vi "Error Manager (Main).vi"(8 "Error In":errorcluster, 11 "Settings Filepath":path) -> (0 "Error Out":errorcluster)   [LabVIEW 2016, in "Error Manager.lvlib"]
doc: "This is the main VI of the Error Manager module.\n\nThe Error Manager is a stand-alone, asynchronous LabVIEW module that can help log LabVIEW errors to file, display error details to the user, and display the chronological or inverse-chronological list of errors that occurred since the module started. The module is framework-agnostic, reusable from project to project, and can keep working even when being \"spammed\" with many instances of the same error (spam protection functionality). Using the Error Manager in a new application helps ensure out-of-the-box robust and reliable error handling.\n\nCopyright (c) 2023, Robusto Systems Ltd (UK)"
uses:
  Error Manager.lvlib
  <vilib>/Utility/error.llb/DialogType.ctl
  Private VIs/Read-Unread Status (enum).ctl
  Private VIs/Reported Error (cluster).ctl
  Multi-Column Listbox/MCL.lvclass
  Error Log/Error Log.lvclass
  Display Order Combo Box/Display Order Combo Box.lvclass
  Queues/MHL Queue/MHL Queue.lvclass
  Queues/MHL Queue/Command (enum).ctl
  Private VIs/Error in current one-second interval (cluster).ctl
  Queues/Log To File Loop Queue/Log To File Loop Queue.lvclass
  Queues/Log To File Loop Queue/Command (enum).ctl
  Error Log/Error Type (enum).ctl
  Error Log/Error to be logged (cluster).ctl
  Queues/New Error Window Loop Queue/Error Window Loop Queue.lvclass
  Queues/New Error Window Loop Queue/Command (enum).ctl
  Error Display Window/Error Display Window.lvclass
  Error Display Window/Error Details (cluster).ctl
  Private VIs/GUI Object References (cluster).ctl
  Mark Selected Errors As Read Button/Mark Selected Errors As Read Button.lvclass
  Mark All Errors As Read Button/Mark All Errors As Read Button.lvclass
  Settings/Settings.lvclass
  Public API VIs/Show Error Window Instruction (enum).ctl
panel:
  out "Module Init Timestamp":timestamp
  out "Read Settings Error":errorcluster
  out "Are All Errors Read?":bool
  out "MCL NewVal":i32[](array[numeric])
  in  "Mark All Errors As Read":bool
  in  "Mark Selected Errors As Read":bool
  out "Metronome Loop iteration":i32
  out "\"New Error Window\" Loop iteration":i32
  out "\"Log to File\" Loop iteration":i32
  out "\"Handle Error\" Error":errorcluster
  in  "Sizing Tool":bool
  in  "Display Order ComboBox":string(combo) caption="Display Order"
  out "Close Module Error":errorcluster
  in  "Open Error Logs Folder":bool
  in  "Open Error Log in Notepad":bool
  out "Error Log Filepath":string
  out "Full Error Message":string caption="Error Message Of Selected Error"
  in  "MCL":i32[](listbox) caption="Errors"
  out "Close Module?":bool
  out "EHL iteration":i32
  out "MHL iteration":i32
  out "Initialisation Error":errorcluster
  # "Error Manager\nThis is the main VI of the Error Manager module."
  # "The region below is invisible to the user. For developer use only."
  # "Input\nInputs to the VI"
  # "Development\ncontrols/indicators useful for development and testing, but which are not outputs of the VI"
  # "Output\nOutputs of the VI"
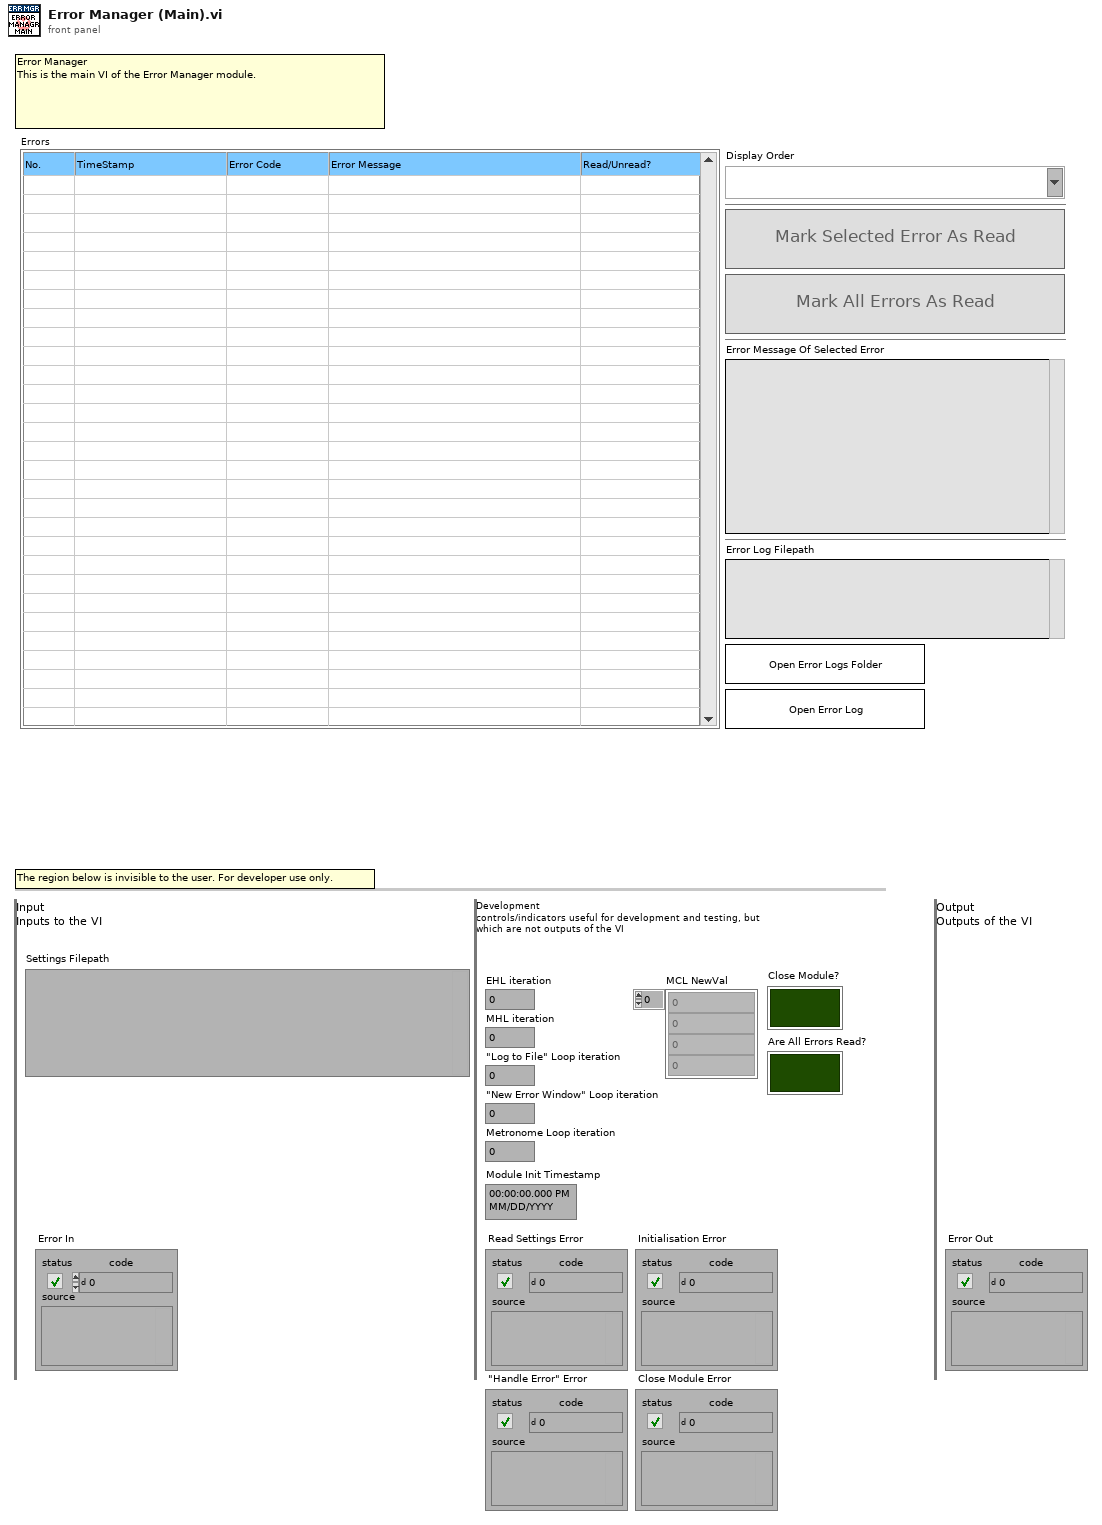
[diagram p1: front panel]
types:
  T1 = typedef "Error Manager.lvlib/MHL Queue.lvclass/Command (enum).ctl" = enum16{"Init Module", "Close Module", "Internal Error", "Create Error Log File", "Show Front Panel", "Handle Error", "Refresh MCL", "MCL Value Change", "Change Display Order", "One-Second Interval Expired", "Mark Selected Errors As Read", "Mark All Errors As Read", "Refresh Button State - MSEAR", "Refresh Button State - MAEAR"}
  T2 = typedef "Error Manager.lvlib/Error Window Loop Queue.lvclass/Command (enum).ctl" = enum16{"Init Loop", "Close Loop", "Show Error Window"}
  T3 = typedef "Error Manager.lvlib/Log To File Loop Queue.lvclass/Command (enum).ctl" = enum16{"Init Loop", "Close Loop", "Log Error"}
  T4 = typedef "Error Manager.lvlib/Read-Unread Status (enum).ctl" = enum16{"Unread", "Read"}
  T5 = typedef "Error Manager.lvlib/GUI Object References (cluster).ctl" = cluster{"MCL":refnum<vi>, "Display Order ComboBox":refnum<vi>, "Mark Selected Errors As Read":refnum<vi>, "Mark All Errors As Read":refnum<vi>, "Full Error Message":refnum<vi>, "Error Log Filepath":refnum<vi>, "Open Error Logs Folder":refnum<vi>, "Open Error Log in Notepad":refnum<vi>}
  T6 = typedef "Error Manager.lvlib/Module Data (cluster).ctl" = cluster{"GUI Object References":T5, "Total no. of errors reported":i32, "Total no. of errors handled":i32, "Handled Errors (chronological order)":T7[], "Display Order":T8, "Errors in current one-second interval":T9[], "Module Init Timestamp":timestamp, "Module Close Timestamp":timestamp}
  T7 = typedef "Error Manager.lvlib/Handled Error (cluster).ctl" = cluster{"Error Number":i32, "Timestamp":timestamp, "Error code":i32, "Error message":string, "Read-Unread Status":T4}
  T8 = typedef "Error Manager.lvlib/Display Order (enum).ctl" = enum16{"Most Recent First (inverse-chronological)", "Oldest First (chronological)"}
  T9 = typedef "Error Manager.lvlib/Error in current one-second interval (cluster).ctl" = cluster{"Error code":i32, "No. of times error reported":u32, "No. of times error handled":u32}
  T10 = typedef "Error Manager.lvlib/Settings.lvclass/Error_Log_Setting (enum).ctl" = enum16{"Log Full Error Details", "Log Error Codes Only", "Do Not Log"}
  T11 = typedef "Error Manager.lvlib/Settings.lvclass/Window_Behaviour (enum).ctl" = enum16{"Default", "Floating", "Modal"}
  T12 = typedef "Error Manager.lvlib/Reported Error (cluster).ctl" = cluster{"Error Timestamp":timestamp, "Error Code":i32, "Error message":string, "Show Error Window?":T13}
  T13 = typedef "Error Manager.lvlib/Show Error Window Instruction (enum).ctl" = enum16{"Use Default Setting", "Show", "Do Not Show"}
  T14 = typedef "Error Manager.lvlib/Error Log.lvclass/Error to be logged (cluster).ctl" = cluster{"Error Type":T15, "Error Number":i32, "Error Timestamp":timestamp, "Error code":i32, "Error message":string}
  T15 = typedef "Error Manager.lvlib/Error Log.lvclass/Error Type (enum).ctl" = enum16{"New", "Identical to last logged error"}
  T16 = typedef "Error Manager.lvlib/Settings.lvclass/Show_Error_Window_Default (enum).ctl" = enum16{"Show For All Errors", "Show For New Errors", "Show For New Error Codes", "Do Not Show"}
  T17 = typedef "Error Manager.lvlib/Error Display Window.lvclass/Error Details (cluster).ctl" = cluster{"Error Code":i32, "Error Message":string, "Error Timestamp":timestamp}
  T18 = typedef "DialogType.ctl" = u16
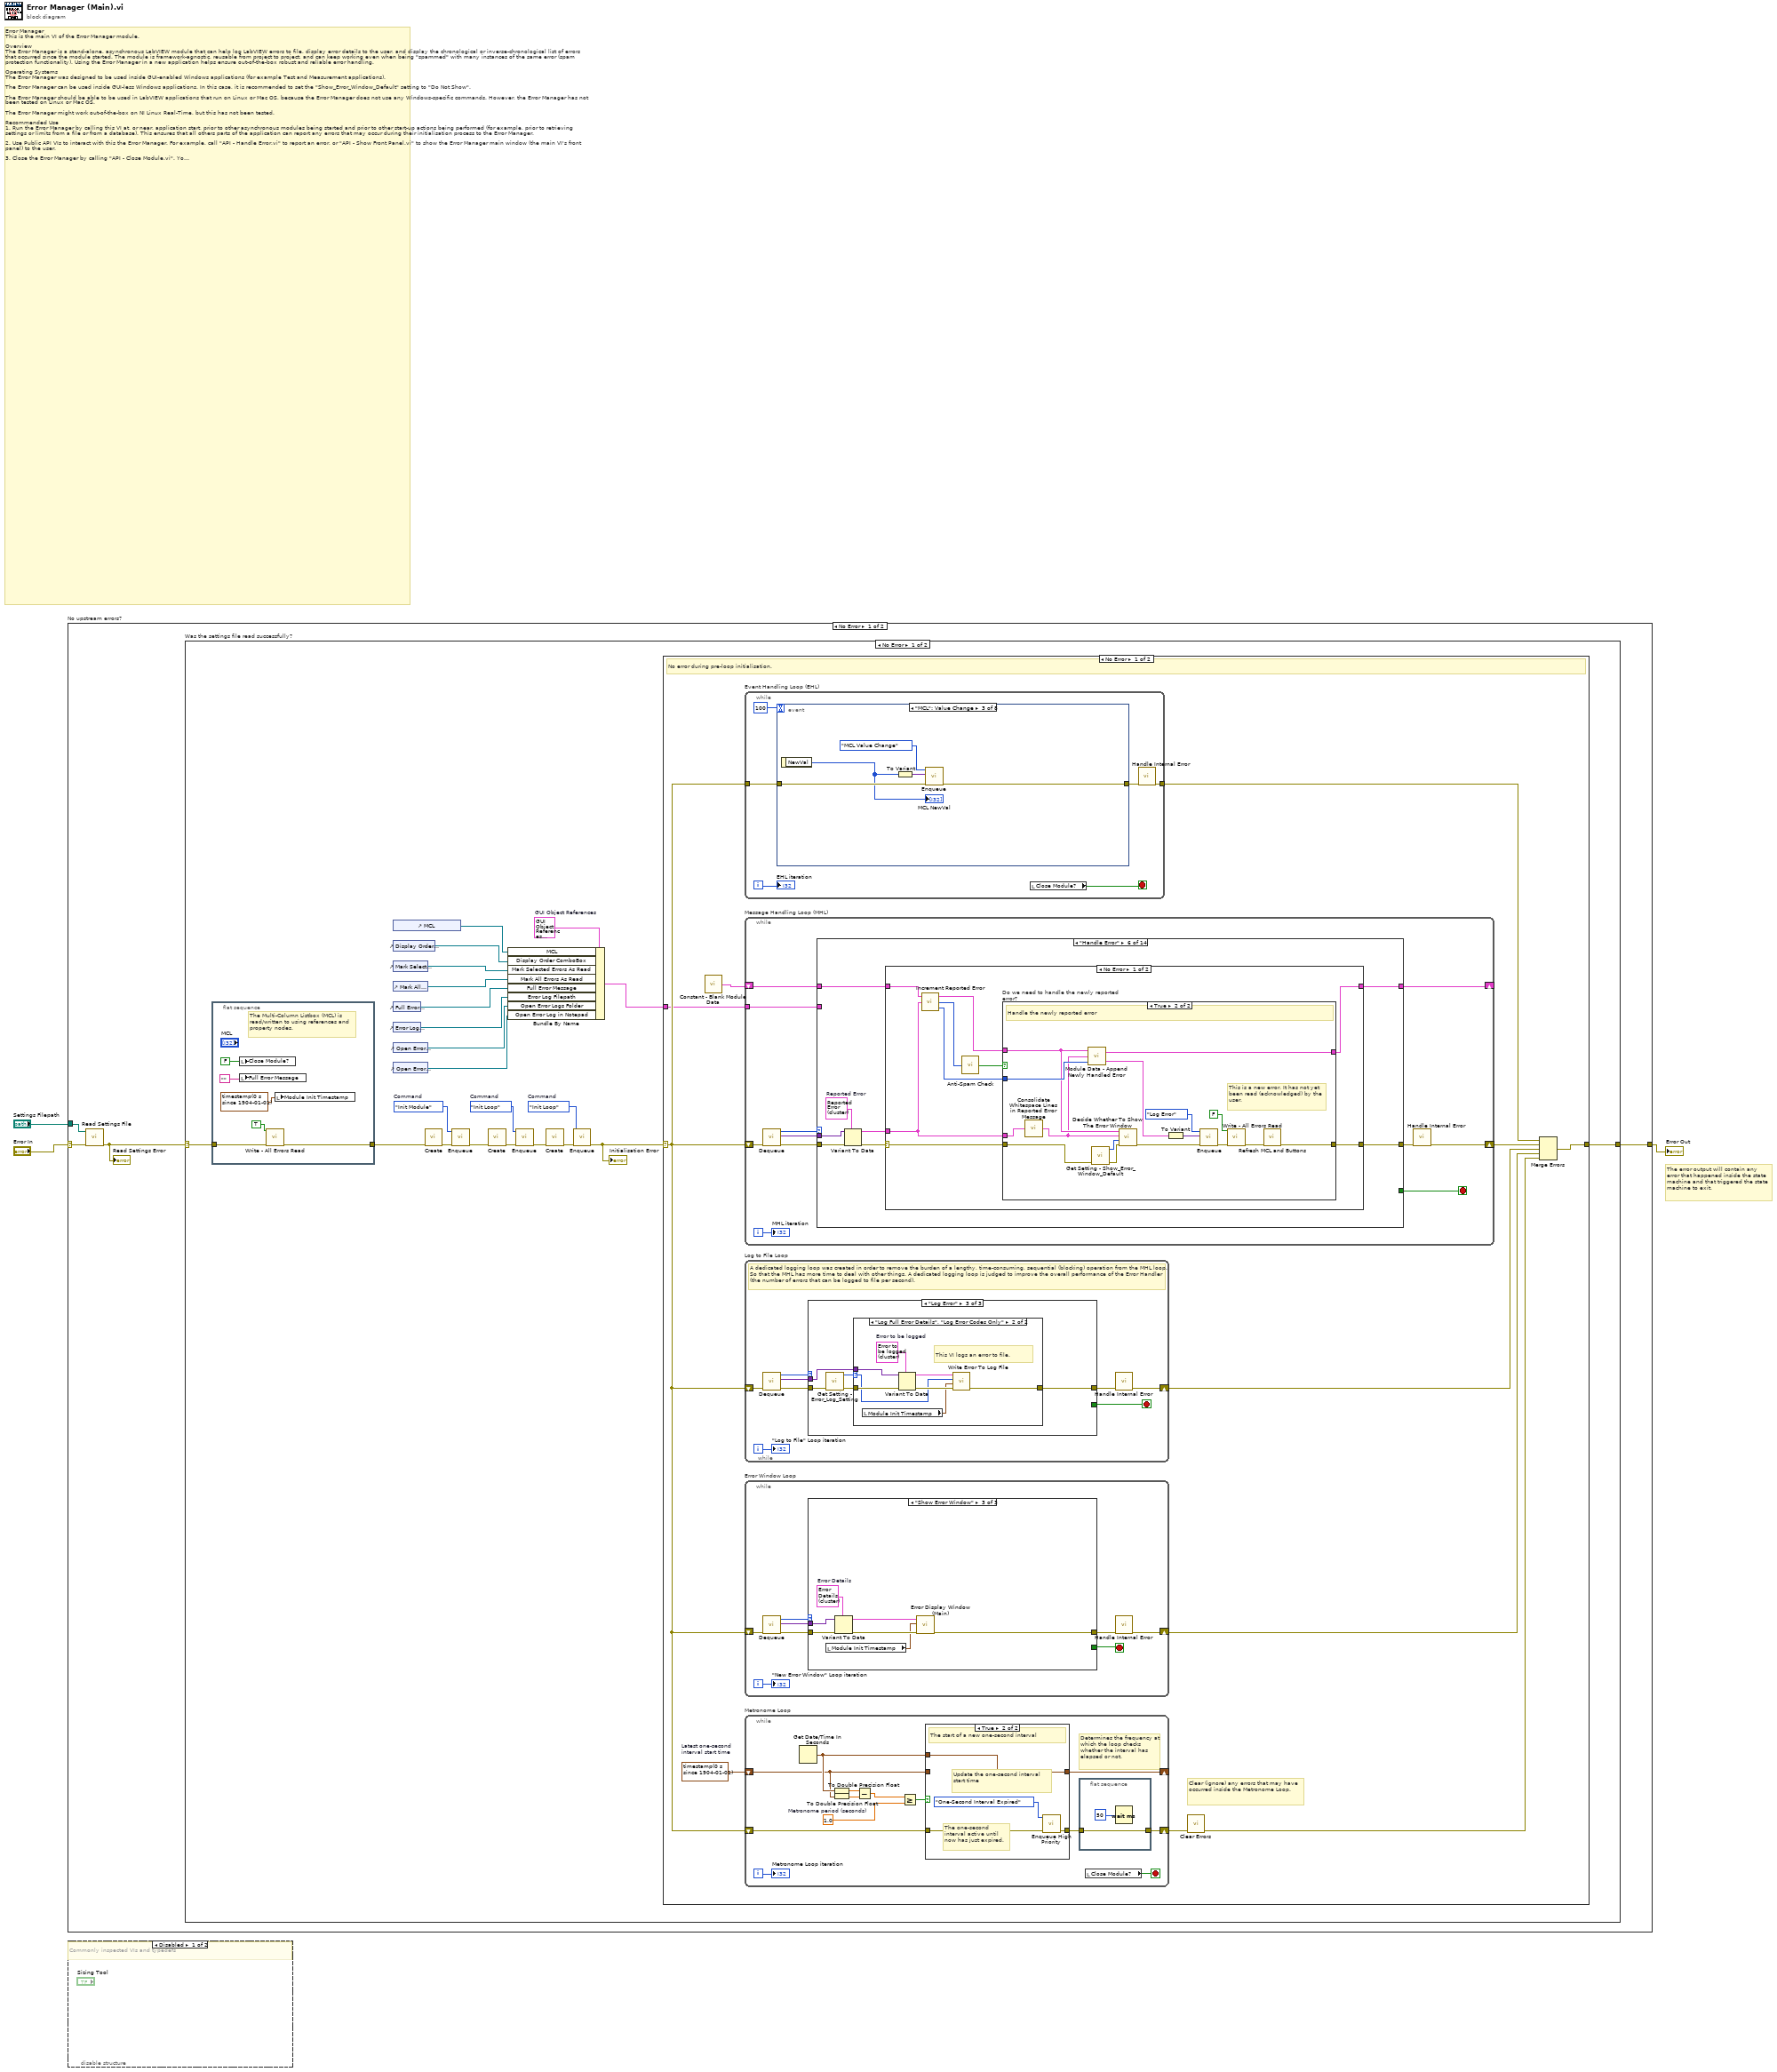
[diagram p0: block diagram]
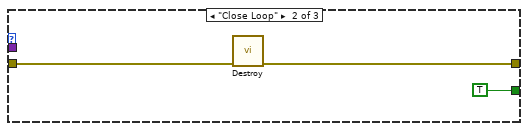
[diagram p3: hidden frame]
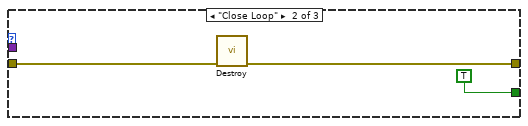
[diagram p5: hidden frame]
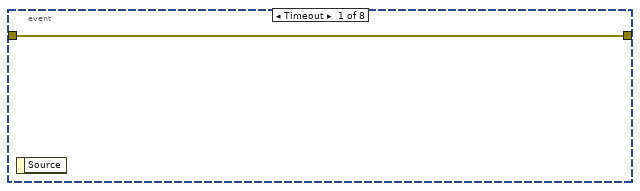
[diagram p7: hidden frame]
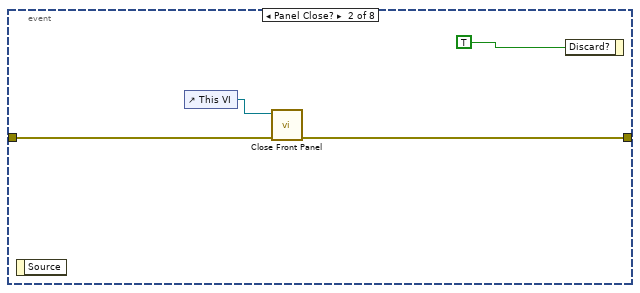
[diagram p8: hidden frame]
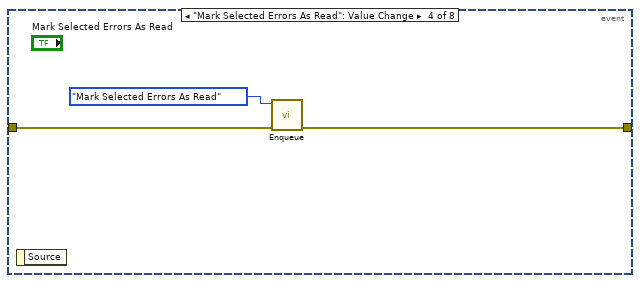
[diagram p9: hidden frame]
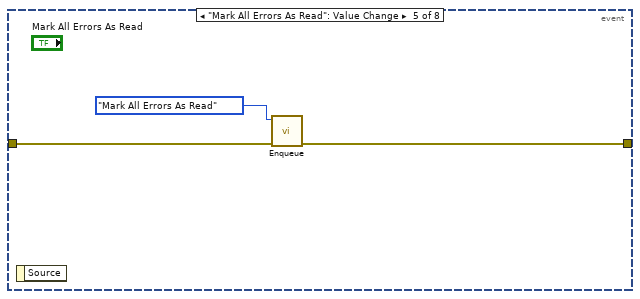
[diagram p10: hidden frame]
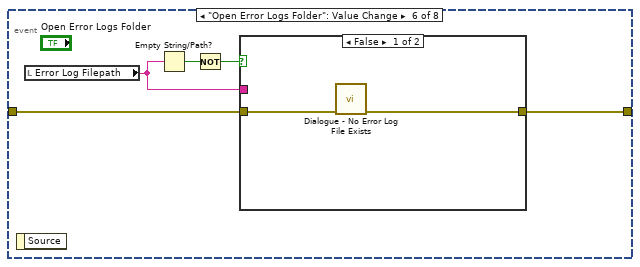
[diagram p11: hidden frame]
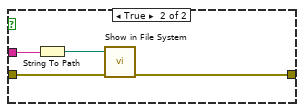
[diagram p12: hidden frame]
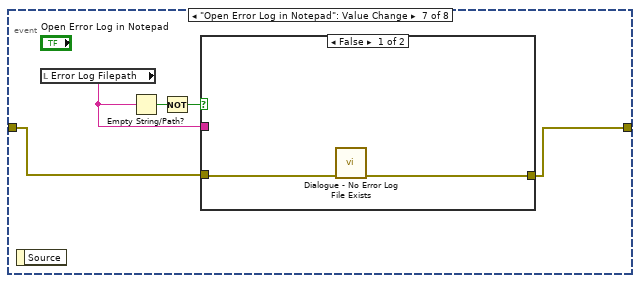
[diagram p13: hidden frame]
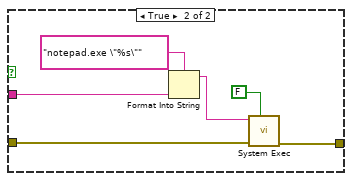
[diagram p14: hidden frame]
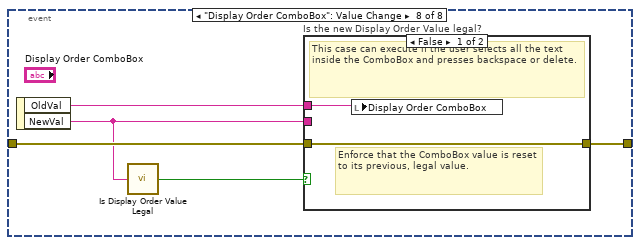
[diagram p15: hidden frame]
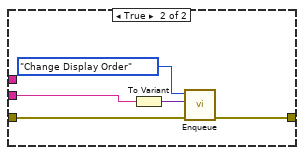
[diagram p16: hidden frame]
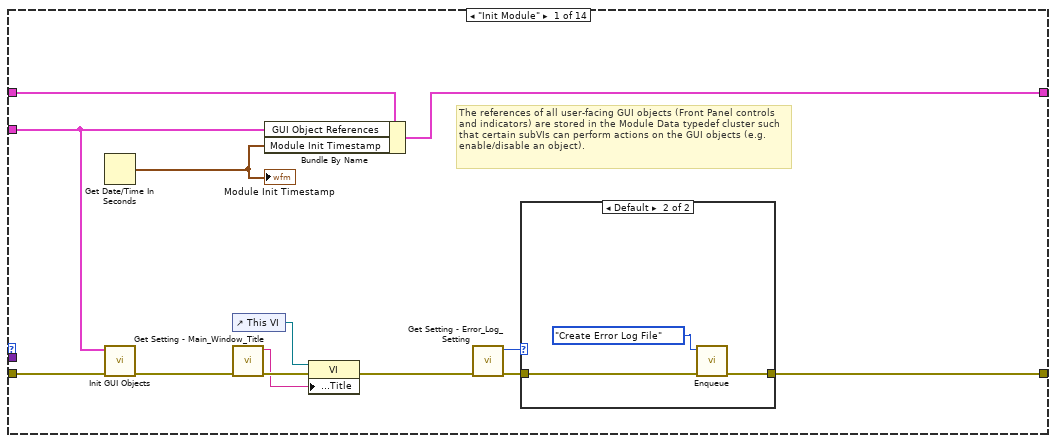
[diagram p17: hidden frame]
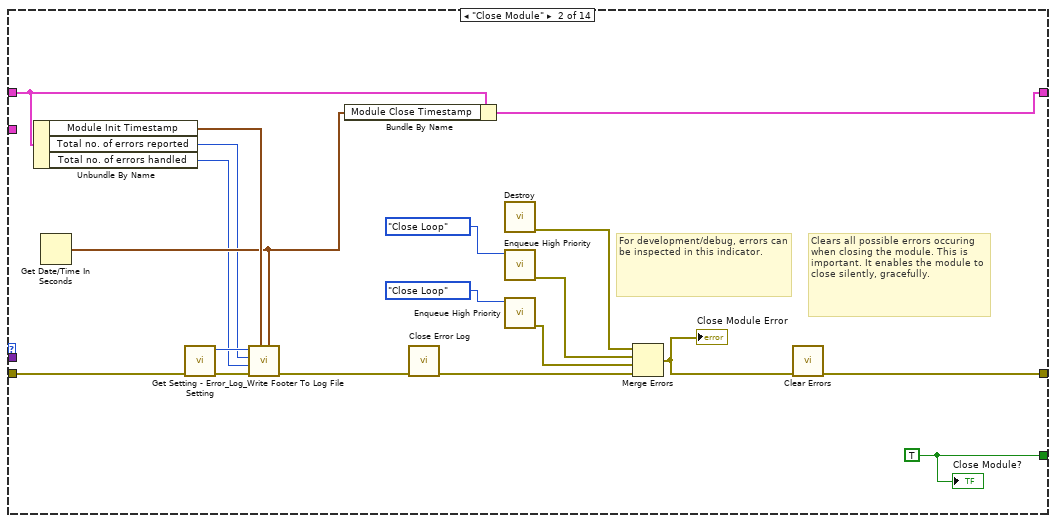
[diagram p19: hidden frame]
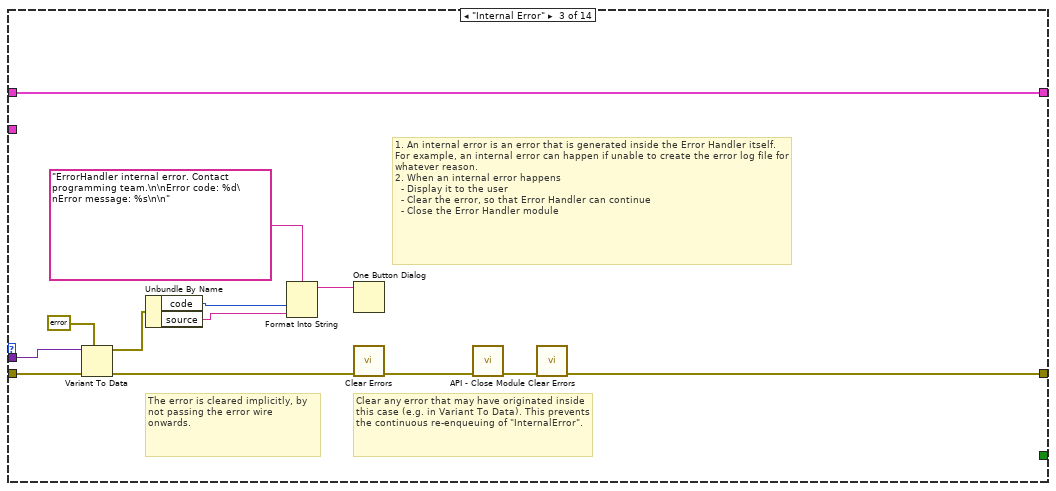
[diagram p20: hidden frame]
diagram:
  # "Error Manager\nThis is the main VI of the Error Manager module.\n\nOverview\nThe Error Manager is a stand-alone, asynchronous LabVIEW module that can help log LabVIEW errors to file, display error details to the user, and display the chronological or inverse-chronological list of errors that occurred since the module started. The module is framework-agnostic, reusable from project to project, and can keep working even when being \"spammed\" with many instances of the same error (spam protection functionality). Using the Error Manager in a new application helps ensure out-of-the-box robust and reliable error handling.\n\nOperating Systems\nThe Error Manager was designed to be used inside GUI-enabled Windows applications (for example Test and Measurement applications).\n\nThe Error Manager can be used inside GUI-less Windows applications. In this case, it is recommended to set the \"Show_Error_Window_Default\" setting to \"Do Not Show\".\n\nThe Error Manager should be able to be used in LabVIEW applications that run on Linux or Mac OS, because the Error Manager does not use any Windows-specific commands. However, the Error Manager has not been tested on Linux or Mac OS.\n\nThe Error Manager might work out-of-the-box on NI Linux Real-Time, but this has not been tested.\n\nRecommended Use\n1. Run the Error Manager by calling this VI at, or near, application start, prior to other asynchronous modules being started and prior to other start-up actions being performed (for example, prior to retrieving settings or limits from a file or from a database). This ensures that all others parts of the application can report any errors that may occur during their initialisation process to the Error Manager.\n\n2. Use Public API VIs to interact with this the Error Manager. For example, call \"API - Handle Error.vi\" to report an error, or \"API - Show Front Panel.vi\" to show the Error Manager main window (the main VI's front panel) to the user.\n\n3. Close the Error Manager by calling \"API - Close Module.vi\". You can close the Error Manager module at any time you like, but it is recommended to close Error Manager during app shutdown, after all other shutdown operations have been completed (for example, after all other asynchronous modules have been stopped). This enables the Error Manager to log any errors that may occur during app shutdown.\n\nPublic GitHub Repository: https://github.com/RobustoSystems/ErrorManager \n\nSuggestions\nPlease email us at engineering@robustosystems.com with any bug reports or suggestions. Alternatively, feel free to create a new issue in the public GitHub repository.\n\nEULA\nThe Error Manager is free and open-source, and is published under the MIT license, which is one of the most permissive types of licenses. You can use the Error Manager inside commercial, closed-source applications.\n\nMIT License\n\nCopyright (c) 2023, Robusto Systems Ltd (UK)\n\nPermission is hereby granted, free of charge, to any person obtaining a copy\nof this software and associated documentation files (the \"Software\"), to deal\nin the Software without restriction, including without limitation the rights\nto use, copy, modify, merge, publish, distribute, sublicense, and/or sell\ncopies of the Software, and to permit persons to whom the Software is\nfurnished to do so, subject to the following conditions:\n\nThe above copyright notice and this permission notice shall be included in all\ncopies or substantial portions of the Software.\n\nTHE SOFTWARE IS PROVIDED \"AS IS\", WITHOUT WARRANTY OF ANY KIND, EXPRESS OR\nIMPLIED, INCLUDING BUT NOT LIMITED TO THE WARRANTIES OF MERCHANTABILITY,\nFITNESS FOR A PARTICULAR PURPOSE AND NONINFRINGEMENT. IN NO EVENT SHALL THE\nAUTHORS OR COPYRIGHT HOLDERS BE LIABLE FOR ANY CLAIM, DAMAGES OR OTHER\nLIABILITY, WHETHER IN AN ACTION OF CONTRACT, TORT OR OTHERWISE, ARISING FROM,\nOUT OF OR IN CONNECTION WITH THE SOFTWARE OR THE USE OR OTHER DEALINGS IN THE\nSOFTWARE."
  # "The error output will contain any error that happened inside the state machine and that triggered the state machine to exit."
  n1 = case "No upstream errors?" shown="No Error" "Error In" {
    selector: "Error In" -> [w6 w419]
    tunnel: [w7 w419] -> w3
    tunnel: "Settings Filepath" -> [w5 _]
    frame No Error {
      n2 = call "Read Settings File.vi"("error in (no error)"=w6, "Settings Filepath"=w5) -> ("error out"=w4:errorcluster)  [unwired: 9 in]
      "Read Settings Error" <- w4
      n3 = case "Was the settings file read successfully?" shown="No Error" w4 {
        selector: w4 -> [w8 w417]
        tunnel: [w29 w416] -> w7
        frame No Error {
          w18 = T5 {"MCL"=refnum, "Display Order ComboBox"=refnum, "Mark Selected Errors As Read"=refnum, "Mark All Errors As Read"=refnum, "Full Error Message"=refnum, "Error Log Filepath"=refnum, "Open Error Logs Folder"=refnum, "Open Error Log in Notepad"=refnum}  # GUI Object References
          w20 = Command_(enum)."Init Loop"  # Command
          w23 = Command_(enum)."Init Loop"  # Command
          w26 = Command_(enum)."Init Module"  # Command
          n4 = flat-sequence {
            tunnel: [w34] -> w19
            tunnel: w8 -> [w33]
            frame #0 {
              # "The Multi-Column Listbox (MCL) is read/written to using references and property nodes."
              n5 = local write "Close Module?"(FALSE ("Close module?")) -> ()
              n6 = local write "Full Error Message"("") -> ()
              n7 = call "Write - All Errors Read.vi"("error in (no error)"=w33, "All Errors Read?"=TRUE) -> ("error out"=w34:errorcluster)  [unwired: 9 in]
              n8 = local write "Module Init Timestamp"(timestamp(0 s since 1904-01-01) ("Module Init Timestamp")) -> ()
            }
          }
          n9 = control-ref of="MCL"() -> (w17:refnum<vi>)
          n10 = control-ref of="Display Order ComboBox"() -> (w16:refnum<vi>)
          n11 = control-ref of="Mark Selected Errors As Read"() -> (w15:refnum<vi>)
          n12 = control-ref of="Mark All Errors As Read"() -> (w14:refnum<vi>)
          n13 = control-ref of="Full Error Message"() -> (w13:refnum<vi>)
          n14 = control-ref of="Error Log Filepath"() -> (w12:refnum<vi>)
          n15 = control-ref of="Open Error Logs Folder"() -> (w11:refnum<vi>)
          n16 = control-ref of="Open Error Log in Notepad"() -> (w10:refnum<vi>)
          n17 = call "Create.vi"("error in (no error)"=w19) -> ("error out"=w28:errorcluster)  [unwired: 10 in]
          n18 = call "Enqueue.vi"("error in (no error)"=w28, "Command"=w26) -> ("error out"=w27:errorcluster)  [unwired: 9 in]
          n19 = call "Create.vi"("error in (no error)"=w27) -> ("error out"=w25:errorcluster)  [unwired: 10 in]
          n20 = Bundle By Name(cluster=w18, "MCL"=w17, "Display Order ComboBox"=w16, "Mark Selected Errors As Read"=w15, "Mark All Errors As Read"=w14, "Full Error Message"=w13, "Error Log Filepath"=w12, "Open Error Logs Folder"=w11, "Open Error Log in Notepad"=w10) -> (w9:T5)
          n21 = call "Enqueue.vi"("error in (no error)"=w25, "Command"=w23) -> ("error out"=w24:errorcluster)  [unwired: 9 in]
          n22 = call "Create.vi"("error in (no error)"=w24) -> ("error out"=w22:errorcluster)  [unwired: 10 in]
          n23 = call "Enqueue.vi"("error in (no error)"=w22, "Command"=w20) -> ("error out"=w21:errorcluster)  [unwired: 9 in]
          "Initialisation Error" <- w21
          n24 = case shown="No Error" w21 {
            selector: w21 -> [w39 w415]
            tunnel: [w45 w414] -> w29
            tunnel: w9 -> [w36 _]
            frame No Error {
              w43 = timestamp(0 s since 1904-01-01)  # Latest one-second interval start time
              # "Clear (ignore) any errors that may have occurred inside the Metronome Loop."
              # "No error during pre-loop initialisation."
              n25 = call "Constant - Blank Module Data.vi"() -> ("Blank Module Data"=w41:T6)
              n26 = while "Event Handling Loop (EHL)" {
                tunnel: w39 -> [w94]
                tunnel: [w92] -> w44
                i -> [w97]
                stop <- w95 stop-if-true
                n27 = event shown="[2] \"MCL\": Value Change" {
                  selector: _ -> [_ _ _ _ _ _ _ _]
                  dyn-events: _ -> [_ _ _ _ _ _ _ _]
                  timeout: 100 -> [_ _ _ _ _ _ _ _]
                  tunnel: w94 -> [w98 w100 w107 w110 w113 w115 w126 w142]
                  tunnel: [w98 w99 w106 w109 w112 w114 w125 w141] -> w93
                  event Timeout {
                    n28 = event-data() -> ()  [unwired: 1 in, 1 out]
                  }
                  event Panel Close? {
                    n29 = event-data() -> ()  [unwired: 1 in, 1 out]
                    n30 = control-ref of="This VI"() -> (w101:refnum<vi>)
                    n31 = call "Close Front Panel.vi"("Error In"=w100, "VI Reference"=w101) -> ("Error Out"=w99:errorcluster)  [unwired: 9 in]
                    n32 = event-data("Discard?"=TRUE) -> ()  [unwired: 1 in, 1 out]
                  }
                  event "MCL": Value Change {
                    n33 = event-data() -> ("NewVal"=w104:i32[])  [unwired: 1 in]
                    "MCL NewVal" <- w104
                    n34 = To Variant(anything=w104) -> (Variant=w103:variant)
                    n35 = call "Enqueue.vi"("error in (no error)"=w107, "Data"=w103, "Command"=Command_(enum)."MCL Value Change") -> ("error out"=w106:errorcluster)  [unwired: 8 in]
                  }
                  event "Mark Selected Errors As Read": Value Change {
                    n36 = event-data() -> ()  [unwired: 1 in, 1 out]
                    n37 = call "Enqueue.vi"("error in (no error)"=w110, "Command"=Command_(enum)."Mark Selected Errors As Read") -> ("error out"=w109:errorcluster)  [unwired: 9 in]
                  }
                  event "Mark All Errors As Read": Value Change {
                    n38 = event-data() -> ()  [unwired: 1 in, 1 out]
                    n39 = call "Enqueue.vi"("error in (no error)"=w113, "Command"=Command_(enum)."Mark All Errors As Read") -> ("error out"=w112:errorcluster)  [unwired: 9 in]
                  }
                  event "Open Error Logs Folder": Value Change {
                    n40 = event-data() -> ()  [unwired: 1 in, 1 out]
                    n41 = local read "Error Log Filepath"() -> (w116:string)
                    n42 = Empty String/Path?(string/path=w116) -> (empty?=w118:bool)
                    n43 = Not(x=w118) -> (.not. x?=w117:bool)
                    n44 = case shown="False" w117 {
                      tunnel: w116 -> [_ w123]
                      tunnel: w115 -> [w119 w122]
                      tunnel: [w120 w121] -> w114
                      frame False {
                        n45 = call "Dialogue - No Error Log File Exists.vi"("error in (no error)"=w119) -> ("error out"=w120:errorcluster)  [unwired: 10 in]
                      }
                      frame True {
                        n46 = String To Path(string=w123) -> (path=w124:path)
                        n47 = call <vilib>:"Show in File System.vi"("error in (no error)"=w122, "file or directory path"=w124) -> ("error out"=w121:errorcluster)  [unwired: 9 in]
                      }
                    }
                  }
                  event "Open Error Log in Notepad": Value Change {
                    n48 = event-data() -> ()  [unwired: 1 in, 1 out]
                    n49 = local read "Error Log Filepath"() -> (w127:string)
                    n50 = Empty String/Path?(string/path=w127) -> (empty?=w128:bool)
                    n51 = Not(x=w128) -> (.not. x?=w129:bool)
                    n52 = case shown="False" w129 {
                      tunnel: w126 -> [w131 w135]
                      tunnel: [w130 w134] -> w125
                      tunnel: w127 -> [_ w133]
                      frame False {
                        n53 = call "Dialogue - No Error Log File Exists.vi"("error in (no error)"=w131) -> ("error out"=w130:errorcluster)  [unwired: 10 in]
                      }
                      frame True {
                        n54 = Format Into String(format string="notepad.exe \"%s\"", w133) -> (resulting string=w136:string)  [unwired: 2 in, 1 out]
                        n55 = call <vilib>:"System Exec.vi"("wait until completion? (T)"=FALSE, "error in (no error)"=w135, "command line"=w136) -> ("error out"=w134:errorcluster)  [unwired: 5 in, 3 out]
                      }
                    }
                  }
                  event "Display Order ComboBox": Value Change {
                    n56 = event-data() -> ("OldVal"=w138:string, "NewVal"=w140:string)  [unwired: 1 in]
                    n57 = call "Is Display Order Value Legal.vi"("New Display Order Value"=w140) -> ("Is Display Order Value Legal?"=w139:bool)
                    n58 = case "Is the new Display Order Value legal?" shown="False" w139 {
                      tunnel: w142 -> [w144 w149]
                      tunnel: [w144 w148] -> w141
                      tunnel: w140 -> [_ w145]
                      tunnel: w138 -> [w143 _]
                      frame False {
                        # "Enforce that the ComboBox value is reset to its previous, legal value."
                        # "This case can execute if the user selects all the text inside the ComboBox and presses backspace or delete."
                        n59 = local write "Display Order ComboBox"(w143) -> ()
                      }
                      frame True {
                        n60 = To Variant(anything=w145) -> (Variant=w147:variant)
                        n61 = call "Enqueue.vi"("error in (no error)"=w149, "Data"=w147, "Command"=Command_(enum)."Change Display Order") -> ("error out"=w148:errorcluster)  [unwired: 8 in]
                      }
                    }
                  }
                }
                n62 = local read "Close Module?"() -> (w95:bool)
                n63 = call "Handle Internal Error.vi"("error in (no error)"=w93) -> ("error out"=w92:errorcluster)  [unwired: 10 in]
                "EHL iteration" <- w97
              }
              n64 = while "Message Handling Loop (MHL)" {
                shift-right: [w154] -> w46
                shift-left: w39 -> [w158]
                shift-right: [w156] -> _
                shift-left: w41 -> [w151]
                tunnel: w36 -> [w150]
                i -> [w157]
                stop <- w160 stop-if-true
                n65 = call "Dequeue.vi"("error in (no error)"=w158) -> ("error out"=w159:errorcluster, "Data"=w152:variant, "Command"=w153:T1)  [unwired: 8 in]
                n66 = case shown="\"Handle Error\"" w153 {
                  tunnel: w159 -> [w169 w185 w206 w213 w229 w243 w278 w291 w310 w323 w338 w352 w381 w391]
                  tunnel: [w173 w194 w197 w215 w234 w240 w277 w284 w305 w322 w334 w342 w379 w389] -> w155
                  tunnel: [_ w195 _ _ _ _ _ _ _ _ _ _ _ _] -> w160
                  tunnel: w152 -> [_ _ w204 _ _ w241 _ w287 w301 _ _ _ _ _]
                  tunnel: w151 -> [w168 w182 w202 w211 w235 w237 w281 w290 w303 w319 w336 w349 w383 w388]
                  tunnel: [w167 w183 w202 w211 w235 w238 w281 w290 w304 w320 w335 w348 w383 w388] -> w156
                  tunnel: w150 -> [w166 _ _ _ _ _ _ _ _ _ _ _ _ _]
                  frame "Init Module" {
                    # "The references of all user-facing GUI objects (Front Panel controls and indicators) are stored in the Module Data typedef cluster such that certain subVIs can perform actions on the GUI objects (e.g. enable/disable an object)."
                    n67 = Get Date/Time In Seconds() -> (seconds since 1Jan1904=w161:timestamp)
                    "Module Init Timestamp" <- w161
                    n68 = call "Init GUI Objects.vi"("Error In"=w169, "GUI Object References"=w166) -> ("Error Out"=w170:errorcluster)  [unwired: 9 in]
                    n69 = control-ref of="This VI"() -> (w171:refnum<vi>)
                    n70 = call "Get Setting - Main_Window_Title.vi"("Error In"=w170) -> ("Error Out"=w165:errorcluster, "Main_Window_Title"=w164:string)  [unwired: 9 in]
                    n71 = Bundle By Name(cluster=w168, "GUI Object References"=w166, "Module Init Timestamp"=w161) -> (w167:T6)
                    n72 = property class="VI"(reference=w171, error in=w165, "Front Panel.Title"=w164) -> (error out=w172:errorcluster)  [unwired: 1 out]
                    n73 = call "Get Setting - Error_Log_Setting.vi"("Error In"=w172) -> ("Error Out"=w163:errorcluster, "Error_Log_Setting"=w162:T10)  [unwired: 9 in]
                    n74 = case shown="Default" w162 {
                      tunnel: [w174 w177] -> w173
                      tunnel: w163 -> [w174 w175]
                      frame "Do Not Log" {
                        # "Don't create a log file if the setting is set to \"Do Not Log\"."
                      }
                      frame Default {
                        n75 = call "Enqueue.vi"("error in (no error)"=w175, "Command"=Command_(enum)."Create Error Log File") -> ("error out"=w177:errorcluster)  [unwired: 9 in]
                      }
                    }
                  }
                  frame "Close Module" {
                    w195 = TRUE
                    # "For development/debug, errors can be inspected in this indicator."
                    # "Clears all possible errors occuring when closing the module. This is important. It enables the module to close silently, gracefully."
                    n76 = Unbundle By Name(w182) -> ("Module Init Timestamp"=w181:timestamp, "Total no. of errors reported"=w179:i32, "Total no. of errors handled"=w178:i32)
                    n77 = Get Date/Time In Seconds() -> (seconds since 1Jan1904=w180:timestamp)
                    n78 = call "Get Setting - Error_Log_Setting.vi"("Error In"=w185) -> ("Error Out"=w188:errorcluster, "Error_Log_Setting"=w184:T10)  [unwired: 9 in]
                    n79 = call "Write Footer To Log File.vi"("Module Close Timestamp"=w180, "Module Init Timestamp"=w181, "error in (no error)"=w188, "Total no. of errors handled"=w178, "Total no. of errors reported"=w179, "Error_Log_Setting"=w184) -> ("error out"=w187:errorcluster)  [unwired: 5 in]
                    n80 = Bundle By Name(cluster=w182, "Module Close Timestamp"=w180) -> (w183:T6)
                    n81 = call "Close Error Log.vi"("error in (no error)"=w187) -> ("error out"=w186:errorcluster)  [unwired: 10 in]
                    n82 = call "Destroy.vi"() -> ("error out"=w196:errorcluster)  [unwired: 9 in, 2 out]
                    n83 = call "Enqueue High Priority.vi"("Command"=Command_(enum)."Close Loop") -> ("error out"=w191:errorcluster)  [unwired: 10 in]
                    n84 = call "Enqueue High Priority.vi"("Command"=Command_(enum)."Close Loop") -> ("error out"=w190:errorcluster)  [unwired: 10 in]
                    n85 = Merge Errors(w196, w191, w190, w186) -> (w193:errorcluster)
                    "Close Module Error" <- w193
                    n86 = call <vilib>:"Clear Errors.vi"("error in (no error)"=w193) -> ("error out"=w194:errorcluster)  [unwired: 5 in, 1 out]
                    "Close Module?" <- w195
                  }
                  frame "Internal Error" {
                    # "The error is cleared implicitly, by not passing the error wire onwards."
                    # "1. An internal error is an error that is generated inside the Error Handler itself. For example, an internal error can happen if unable to create the error log file for whatever reason.\n2. When an internal error happens\n  - Display it to the user\n  - Clear the error, so that Error Handler can continue\n  - Close the Error Handler module"
                    # "Clear any error that may have originated inside this case (e.g. in Variant To Data). This prevents the continuous re-enqueuing of \"InternalError\"."
                    n87 = Variant To Data(error in=w206, type=errorcluster {"status"=FALSE, "code"=0, "source"=""} ("error constant"), Variant=w204) -> (data=w201:errorcluster, error out=w203:errorcluster)
                    n88 = Unbundle By Name(w201) -> ("code"=w207:i32, "source"=w200:string)
                    n89 = Format Into String(format string="ErrorHandler internal error. Contact programming team.\n\nError code: %d\nError message: %s\n\n" ("Warning"), w207, w200) -> (resulting string=w208:string)  [unwired: 2 in, 1 out]
                    n90 = One Button Dialog(message=w208) -> ()  [unwired: 1 in, 1 out]
                    n91 = call <vilib>:"Clear Errors.vi"("error in (no error)"=w203) -> ("error out"=w199:errorcluster)  [unwired: 5 in, 1 out]
                    n92 = call "API - Close Module.vi"("error in"=w199) -> ("error out"=w198:errorcluster)  [unwired: 10 in]
                    n93 = call <vilib>:"Clear Errors.vi"("error in (no error)"=w198) -> ("error out"=w197:errorcluster)  [unwired: 5 in, 1 out]
                  }
                  frame "Create Error Log File" {
                    n94 = Unbundle By Name(w211) -> ("Module Init Timestamp"=w210:timestamp)
                    n95 = call "Get Setting - Error_Log_Setting.vi"("Error In"=w213) -> ("Error Out"=w214:errorcluster, "Error_Log_Setting"=w212:T10)  [unwired: 9 in]
                    n96 = case shown="\"Log Full Error Details\", \"Log Error Codes Only\"" w212 {
                      tunnel: [w216 w225] -> w215
                      tunnel: w214 -> [w216 w218]
                      tunnel: w210 -> [_ w217]
                      frame "Do Not Log" {
                        # "Don't create a log file if the setting is set to \"Do Not Log\"."
                      }
                      frame "Log Full Error Details", "Log Error Codes Only" {
                        # "Creates the Error Log file."
                        n97 = call "Get Setting - Error_Log_Folder.vi"("Error In"=w218) -> ("Error Out"=w222:errorcluster, "Error_Log_Folder"=w223:path)  [unwired: 9 in]
                        n98 = call "Get Setting - Application_Name.vi"("Error In"=w222) -> ("Error Out"=w221:errorcluster, "Application_Name"=w220:string)  [unwired: 9 in]
                        n99 = call "Ensure Error Logs Folder Is Valid.vi"("Error In"=w221, "Application Name"=w220, "Error Logs Folder (as provided by calling application)"=w223) -> ("Error Out"=w219:errorcluster, "Error Logs Folder (valid)"=w224:path)  [unwired: 7 in]
                        n100 = call "Create Error Log.vi"("error in (no error)"=w219, "Module Init Timestamp"=w217, "Application Name"=w220, "The folder to store the Error Logs"=w224) -> ("error out"=w225:errorcluster, "Full file path of the Error Log"=w227:path)  [unwired: 6 in]
                        n101 = Path To String(path=w227) -> (string=→"Error Log Filepath":string)
                      }
                    }
                  }
                  frame "Show Front Panel" {
                    w231 = i16 605  # Window Vertical Size (pixels)
                    w232 = i16 1055  # Window Horizontal Size (pixels)
                    # "Displays the front panel window of this VI (the Error Manager Main VI) to the user. This action typically executes when the user presses a button that enables them to view the list of errors that may have occurred in the application up to that point."
                    n102 = call "Get Setting - Main_Window_Behaviour.vi"("Error In"=w229) -> ("Error Out"=w230:errorcluster, "Main_Window_Behaviour"=w228:T11)  [unwired: 9 in]
                    n103 = control-ref of="This VI"() -> (w233:refnum<vi>)
                    n104 = call "Show Front Panel.vi"("Window Vertical Size (pixels)"=w231, "Window Horizontal Size (pixels)"=w232, "Error In"=w230, "Window Behaviour"=w228, "VI Reference"=w233) -> ("Error Out"=w234:errorcluster)  [unwired: 6 in]
                  }
                  frame "Handle Error" {
                    w236 = T12 {"Error Timestamp"=timestamp(0 s since 1904-01-01), "Error Code"=0, "Error message"="", "Show Error Window?"=enum."Use Default Setting"}  # Reported Error
                    n105 = Variant To Data(error in=w243, type=w236, Variant=w241) -> (data=w239:T12, error out=w242:errorcluster)
                    n106 = case shown="No Error" w242 {
                      selector: w242 -> [w251 w271]
                      tunnel: [w250 w273] -> w240
                      tunnel: w239 -> [w247 _]
                      tunnel: [w252 w272] -> w238
                      tunnel: w237 -> [w248 w272]
                      frame No Error {
                        n107 = call "Increment Reported Error.vi"("Newly Reported Error"=w247, "Module Data in"=w248) -> ("Index of the newly reported error in the OSI data structure"=w244:i32, "No. of times this error code was handled in the last second"=w246:u32, "Module Data out (OSI data updated)"=w249:T6)  [unwired: 1 in]
                        n108 = call "Anti-Spam Check.vi"("No. of times the same error code has been handled in current One-Second Interval"=w246) -> ("Need to handle this error?"=w245:bool)
                        n109 = case "Do we need to handle the newly reported error?" shown="True" w245 {
                          tunnel: [w254 w263] -> w252
                          tunnel: w251 -> [w253 w264]
                          tunnel: [w253 w259] -> w250
                          tunnel: w249 -> [w254 w262]
                          tunnel: w247 -> [_ w255]
                          tunnel: w244 -> [_ w269]
                          frame False {
                            # "Do nothing."
                            # "The newly reported error is spam. Don't handle it."
                          }
                          frame True {
                            # "This is a new error. It has not yet been read (acknowledged) by the user."
                            # "Handle the newly reported error"
                            n110 = call "Consolidate Whitespace Lines in Reported Error Message.vi"("Reported Error In"=w255) -> ("Reported Error Out (error message consolidated whitelines)"=w256:T12)
                            n111 = call "Module Data - Append Newly Handled Error.vi"("Index of the newly reported error in the OSI data structure"=w269, "Newly Reported Error"=w256, "Module Data in"=w262) -> ("Error to be logged to file"=w267:T14, "Module Data out (Error appended)"=w263:T6)
                            n112 = call "Get Setting - Show_Error_Window_Default.vi"("Error In"=w264) -> ("Error Out"=w258:errorcluster, "Show_Error_Window_Default"=w257:T16)  [unwired: 9 in]
                            n113 = call "Decide Whether To Show The Error Window.vi"("Error In"=w258, "Show Error Window (Default Setting)"=w257, "Newly Reported Error"=w256, "Module Data in"=w262) -> ("Error Out"=w265:errorcluster)  [unwired: 7 in]
                            n114 = To Variant(anything=w267) -> (Variant=w266:variant)
                            n115 = call "Enqueue.vi"("error in (no error)"=w265, "Data"=w266, "Command"=Command_(enum)."Log Error") -> ("error out"=w261:errorcluster)  [unwired: 8 in]
                            n116 = call "Write - All Errors Read.vi"("error in (no error)"=w261, "All Errors Read?"=FALSE) -> ("error out"=w260:errorcluster)  [unwired: 9 in]
                            n117 = call "Refresh MCL and Buttons.vi"("error in (no error)"=w260) -> ("error out"=w259:errorcluster)  [unwired: 10 in]
                          }
                        }
                      }
                      frame Error {
                        # "This case should never execute. If it executes, fix the issue by making sure that this case is accessed only by calling the \"Handle Error.vi\" API VI."
                        n118 = call <vilib>:"Clear Errors.vi"("error in (no error)"=w271) -> ("error out"=w274:errorcluster)  [unwired: 5 in, 1 out]
                        n119 = call "Throw Error.vi"("error in"=w274, "Error Message"="Assertion. Unable to convert variant to \"Reported Error\" typedef cluster. There is a bug in the code. Contact programming team.") -> ("error out"=w273:errorcluster)  [unwired: 9 in]
                        "\"Handle Error\" Error" <- w271
                      }
                    }
                  }
                  frame "Refresh MCL" {
                    n120 = Unbundle By Name(w281) -> ("Handled Errors (chronological order)"=w279:T7[], "Display Order"=w276:T8)
                    n121 = control-ref of="MCL"() -> (w280:refnum<vi>)
                    n122 = call "Refresh MCL (action).vi"("error in (no error)"=w278, "Display Order"=w276, "Errors To Display"=w279, "MCL Reference"=w280) -> ("error out"=w277:errorcluster)  [unwired: 7 in]
                  }
                  frame "MCL Value Change" {
                    w286 = Command_(enum)."Refresh Button State - MSEAR"  # Command
                    w288 = i32[] []  # MCL New Value
                    n123 = Variant To Data(error in=w291, type=w288, Variant=w287) -> (data=w283:i32[], error out=w285:errorcluster)
                    n124 = Array Size(array=w283) -> (size(s)=w282:i32)
                    n125 = case "How many rows selected?" shown="1" w282 {
                      tunnel: w290 -> [_ w299 _]
                      tunnel: [_ w297 "Multiple errors selected" ("Error message")] -> w289
                      tunnel: w283 -> [_ w292 _]
                      frame 0 {
                        # "Zero rows selected."
                      }
                      frame 1 {
                        # "A single row is selected."
                        n126 = Unbundle By Name(w299) -> ("Handled Errors (chronological order)"=w295:T7[], "Display Order"=w294:T8)
                        n127 = call "Get Handled Errors In Display Order.vi"("Display Order"=w294, "Handled Errors (chronological order)"=w295) -> ("Handled Errors (display order)"=w293:T7[])
                        n128 = Index Array(array=w292) -> (element=w296:i32)  [unwired: 1 in]
                        n129 = Index Array(array=w293, index=w296) -> (element=w298:T7)
                        n130 = Unbundle By Name(w298) -> ("Error message"=w297:string)
                      }
                      frame Default {
                        # "Two or more rows selected."
                      }
                    }
                    "Full Error Message" <- w289
                    n131 = call "Enqueue.vi"("error in (no error)"=w285, "Command"=w286) -> ("error out"=w284:errorcluster)  [unwired: 9 in]
                  }
                  frame "Change Display Order" {
                    # "Raises error if unable to convert string to enum."
                    n132 = Variant To Data(error in=w310, type="", Variant=w301) -> (data=w306:string, error out=w309:errorcluster)
                    n133 = call "Convert String To Enum.vi"("error in (no error)"=w309, "Display Order (ComboBox string)"=w306) -> ("error out"=w307:errorcluster, "Display Order (enum)"=w302:T8)  [unwired: 8 in]
                    n134 = case shown="No Error" w307 {
                      selector: w307 -> [w315 w317]
                      tunnel: [w314 w317] -> w305
                      tunnel: w303 -> [w313 w316]
                      tunnel: [w312 w316] -> w304
                      tunnel: w302 -> [w311 _]
                      frame No Error {
                        # "This case expected to execute always."
                        n135 = Bundle By Name(cluster=w313, "Display Order"=w311) -> (w312:T6)
                        n136 = call "Refresh MCL and Buttons.vi"("error in (no error)"=w315) -> ("error out"=w314:errorcluster)  [unwired: 10 in]
                      }
                      frame Error {
                      }
                    }
                  }
                  frame "One-Second Interval Expired" {
                    w318 = T9[] []  # Blank
                    # "Refresh (clear) the errors accumulated in the last one-second interval."
                    # "This case plays a role in the implementation of 'anti-spam' functionality."
                    n137 = Unbundle By Name(w319) -> ("Errors in current one-second interval"=w321:T9[])
                    n138 = call "Log One-Second Interval Message (if necessary).vi"("error in (no error)"=w323, "Errors in current one-second interval"=w321) -> ("error out"=w322:errorcluster)  [unwired: 9 in]
                    n139 = Bundle By Name(cluster=w319, "Errors in current one-second interval"=w318) -> (w320:T6)
                  }
                  frame "Mark Selected Errors As Read" {
                    n140 = control-ref of="MCL"() -> (w337:refnum<vi>)
                    n141 = Unbundle By Name(w336) -> ("Handled Errors (chronological order)"=w331:T7[], "Display Order"=w329:T8)
                    n142 = call "MCL - Get Selected Rows.vi"("error in (no error)"=w338, "MCL Reference"=w337) -> ("error out"=w325:errorcluster, "Index of Selected Rows"=w333:i32[])  [unwired: 5 in, 3 out]
                    n143 = call "Get Handled Errors In Display Order.vi"("Display Order"=w329, "Handled Errors (chronological order)"=w331) -> ("Handled Errors (display order)"=w330:T7[])
                    n144 = for {
                      tunnel: w333 -> [w341] mode=indexing
                      shift-right: [w340] -> w332
                      shift-left: w330 -> [w339]
                      n145 = call "Mark Selected Error As Read.vi"("MCL Row Index (display drder)"=w341, "Handled Errors (display order)"=w339) -> ("Handled Errors (display order)"=w340:T7[])
                    }
                    n146 = call "Get Handled Errors In Chronological Order.vi"("Display Order"=w329, "Handled Errors (display order)"=w332) -> ("Handled Errors (chronological order)"=w328:T7[])
                    n147 = call "Get Row Indexes Of Unread Errors.vi"("Handled Errors (chronological order)"=w328) -> ("Row Index Of Unread Errors"=w327:i32[])
                    n148 = Empty Array?(array=w327) -> (empty?=w326:bool)
                    "Are All Errors Read?" <- w326
                    n149 = call "Write - All Errors Read.vi"("error in (no error)"=w325, "All Errors Read?"=w326) -> ("error out"=w324:errorcluster)  [unwired: 9 in]
                    n150 = Bundle By Name(cluster=w336, "Handled Errors (chronological order)"=w328) -> (w335:T6)
                    n151 = call "Refresh MCL and Buttons.vi"("error in (no error)"=w324) -> ("error out"=w334:errorcluster)  [unwired: 10 in]
                  }
                  frame "Mark All Errors As Read" {
                    n152 = Unbundle By Name(w349) -> ("Handled Errors (chronological order)"=w344:T7[], "Display Order"=w346:T8)
                    n153 = call "Write - All Errors Read.vi"("error in (no error)"=w352, "All Errors Read?"=TRUE) -> ("error out"=w350:errorcluster)  [unwired: 9 in]
                    n154 = call "Get Row Indexes Of Unread Errors.vi"("Handled Errors (chronological order)"=w344) -> ("Row Index Of Unread Errors"=w345:i32[])
                    n155 = case shown="\"Oldest First (chronological)\"" w346 {
                      tunnel: w350 -> [w357 w369]
                      tunnel: [w356 w368] -> w343
                      tunnel: w345 -> [w355 w366]
                      tunnel: w344 -> [w354 w367]
                      tunnel: [w353 w365] -> w347
                      frame "Oldest First (chronological)" {
                        n156 = for "For each unread error" {
                          shift-right: [w364] -> w356
                          shift-left: w357 -> [w364]
                          tunnel: w355 -> [w358] mode=indexing
                          shift-right: [w359] -> w353
                          shift-left: w354 -> [w361]
                          n157 = Index Array(array=w361, index=w358) -> (element=w360:T7)
                          n158 = Bundle By Name(cluster=w360, "Read-Unread Status"=Read-Unread_Status_(enum)."Read") -> (w362:T7)
                          n159 = Replace Array Subset(array=w361, new element=w362, index=w358) -> (w359:T7[])
                        }
                      }
                      frame "Most Recent First (inverse-chronological)" {
                        n160 = for "For each unread error" {
                          shift-right: [w376] -> w368
                          shift-left: w369 -> [w376]
                          tunnel: w366 -> [w370] mode=indexing
                          shift-right: [w371] -> w365
                          shift-left: w367 -> [w373]
                          n161 = Index Array(array=w373, index=w370) -> (element=w372:T7)
                          n162 = Bundle By Name(cluster=w372, "Read-Unread Status"=Read-Unread_Status_(enum)."Read") -> (w374:T7)
                          n163 = Replace Array Subset(array=w373, new element=w374, index=w370) -> (w371:T7[])
                        }
                      }
                    }
                    n164 = Bundle By Name(cluster=w349, "Handled Errors (chronological order)"=w347) -> (w348:T6)
                    n165 = call "Refresh MCL and Buttons.vi"("error in (no error)"=w343) -> ("error out"=w342:errorcluster)  [unwired: 10 in]
                  }
                  frame "Refresh Button State - MSEAR" {
                    # "MSEAR = \"Mark Selected Errors As Read\" button"
                    n166 = Unbundle By Name(w383) -> ("Handled Errors (chronological order)"=w385:T7[], "Display Order"=w384:T8, "GUI Object References.Mark Selected Errors As Read"=w377:refnum<vi>)
                    n167 = call "Get Handled Errors In Display Order.vi"("Display Order"=w384, "Handled Errors (chronological order)"=w385) -> ("Handled Errors (display order)"=w380:T7[])
                    n168 = local read "MCL"() -> (w378:i32[])
                    n169 = call "Enable or Disable Button.vi"("Error In"=w381, "Mark Selected Errors As Read Button Reference"=w377, "MCL Value"=w378, "Handled Errors (MCL Display Order)"=w380) -> ("Error Out"=w382:errorcluster)  [unwired: 7 in]
                    n170 = call "Set Boolean Text.vi"("Error In"=w382, "Mark Selected Errors As Read Button Reference"=w377, "MCL Value"=w378) -> ("Error Out"=w379:errorcluster)  [unwired: 8 in]
                  }
                  frame "Refresh Button State - MAEAR" {
                    # "MAEAR = \"Mark All Errors As Read\" button"
                    n171 = call "API - Have All Errors Been Read.vi"("error in"=w391) -> ("error out"=w390:errorcluster, "Have All Errors Been Read?"=w386:bool)  [unwired: 9 in]
                    n172 = Unbundle By Name(w388) -> ("GUI Object References.Mark All Errors As Read"=w387:refnum<vi>)
                    n173 = call "Enable or Disable Button.vi"("Error In"=w390, "Have All Errors Been Read?"=w386, "Mark All Errors As Read Button Reference"=w387) -> ("Error Out"=w389:errorcluster)  [unwired: 8 in]
                  }
                }
                n174 = call "Handle Internal Error.vi"("error in (no error)"=w155) -> ("error out"=w154:errorcluster)  [unwired: 10 in]
                "MHL iteration" <- w157
              }
              n175 = while "Log to File Loop" {
                shift-right: [w68] -> w40
                shift-left: w39 -> [w73]
                i -> [w66]
                stop <- w70 stop-if-true
                # "A dedicated logging loop was created in order to remove the burden of a lengthy, time-consuming, sequential (blocking) operation from the MHL loop. So that the MHL has more time to deal with other things. A dedicated logging loop is judged to improve the overall performance of the Error Handler (the number of errors that can be logged to file per second)."
                n176 = call "Dequeue.vi"("error in (no error)"=w73) -> ("error out"=w72:errorcluster, "Data"=w67:variant, "Command"=w71:T3)  [unwired: 8 in]
                n177 = case shown="\"Log Error\"" w71 {
                  tunnel: w72 -> [w74 w75 w81]
                  tunnel: [_ TRUE _] -> w70
                  tunnel: [w74 w76 w82] -> w69
                  tunnel: w67 -> [_ _ w80]
                  frame "Init Loop" {
                  }
                  frame "Close Loop" {
                    n178 = call "Destroy.vi"("error in (no error)"=w75) -> ("error out"=w76:errorcluster)  [unwired: 8 in, 2 out]
                  }
                  frame "Log Error" {
                    n179 = call "Get Setting - Error_Log_Setting.vi"("Error In"=w81) -> ("Error Out"=w79:errorcluster, "Error_Log_Setting"=w78:T10)  [unwired: 9 in]
                    n180 = case shown="\"Log Full Error Details\", \"Log Error Codes Only\"" w78 {
                      selector: w78 -> [_ w85]
                      tunnel: [w83 w91] -> w82
                      tunnel: w80 -> [_ w89]
                      tunnel: w79 -> [w83 w86]
                      frame "Do Not Log" {
                      }
                      frame "Log Full Error Details", "Log Error Codes Only" {
                        w88 = T14 {"Error Type"=enum."New", "Error Number"=0, "Error Timestamp"=timestamp(0 s since 1904-01-01), "Error code"=0, "Error message"=""}  # Error to be logged
                        # "This VI logs an error to file."
                        n181 = local read "Module Init Timestamp"() -> (w84:timestamp)
                        n182 = Variant To Data(error in=w86, type=w88, Variant=w89) -> (data=w87:T14, error out=w90:errorcluster)
                        n183 = call "Write Error To Log File.vi"("error in (no error)"=w90, "Module Init Timestamp"=w84, "Error_Log_Setting"=w85, "Error to be logged"=w87) -> ("error out"=w91:errorcluster)  [unwired: 7 in]
                      }
                    }
                  }
                }
                n184 = call "Handle Internal Error.vi"("error in (no error)"=w69) -> ("error out"=w68:errorcluster)  [unwired: 10 in]
                "\"Log to File\" Loop iteration" <- w66
              }
              n185 = while "Error Window Loop" {
                shift-right: [w52] -> w38
                shift-left: w39 -> [w54]
                i -> [w47]
                stop <- w48 stop-if-true
                n186 = call "Dequeue.vi"("error in (no error)"=w54) -> ("error out"=w51:errorcluster, "Data"=w49:variant, "Command"=w50:T2)  [unwired: 8 in]
                n187 = case shown="\"Show Error Window\"" w50 {
                  tunnel: w51 -> [w55 w56 w65]
                  tunnel: [w55 w57 w64] -> w53
                  tunnel: w49 -> [_ _ w62]
                  tunnel: [_ TRUE _] -> w48
                  frame "Init Loop" {
                  }
                  frame "Close Loop" {
                    n188 = call "Destroy.vi"("error in (no error)"=w56) -> ("error out"=w57:errorcluster)  [unwired: 8 in, 2 out]
                  }
                  frame "Show Error Window" {
                    w61 = T17 {"Error Code"=0, "Error Message"="", "Error Timestamp"=timestamp(0 s since 1904-01-01)}  # Error Details
                    n189 = local read "Module Init Timestamp"() -> (w59:timestamp)
                    n190 = Variant To Data(error in=w65, type=w61, Variant=w62) -> (data=w60:T17, error out=w63:errorcluster)
                    n191 = call "Error Display Window (Main).vi"("Error In"=w63, "Module Init Timestamp"=w59, "Error Details"=w60) -> ("Error Out"=w64:errorcluster)  [unwired: 8 in]
                  }
                }
                n192 = call "Handle Internal Error.vi"("error in (no error)"=w53) -> ("error out"=w52:errorcluster)  [unwired: 10 in]
                "\"New Error Window\" Loop iteration" <- w47
              }
              n193 = while "Metronome Loop" {
                shift-right: [w397] -> _
                shift-left: w43 -> [w396]
                shift-right: [w394] -> w42
                shift-left: w39 -> [w395]
                i -> [w392]
                stop <- w404 stop-if-true
                w400 = 1.0  # Metronome period (seconds)
                # "Determines the frequency at which the loop checks whether the interval has elapsed or not."
                n194 = Get Date/Time In Seconds() -> (seconds since 1Jan1904=w398:timestamp)
                n195 = To Double Precision Float(number=w398) -> (double precision float=w403:dbl)
                n196 = To Double Precision Float(number=w396) -> (double precision float=w402:dbl)
                n197 = Subtract(x=w403, y=w402) -> (x-y=w401:dbl)
                n198 = Greater Or Equal?(x=w401, y=w400) -> (x >= y?=w399:bool)
                n199 = case shown="True" w399 {
                  tunnel: w398 -> [_ w412]
                  tunnel: [w408 w412] -> w397
                  tunnel: w396 -> [w408 _]
                  tunnel: w395 -> [w407 w411]
                  tunnel: [w407 w410] -> w393
                  frame False {
                    # "We are still in the existing one-second interval"
                  }
                  frame True {
                    # "The one-second interval active until now has just expired."
                    # "Update the one-second interval start time"
                    # "The start of a new one-second interval"
                    n200 = call "Enqueue High Priority.vi"("error in (no error)"=w411, "Command"=Command_(enum)."One-Second Interval Expired") -> ("error out"=w410:errorcluster)  [unwired: 9 in]
                  }
                }
                n201 = flat-sequence {
                  tunnel: [w405] -> w394
                  tunnel: w393 -> [w405]
                  frame #0 {
                    n202 = Wait (ms)(milliseconds to wait=u32 50) -> ()  [unwired: 1 out]
                  }
                }
                n203 = local read "Close Module?"() -> (w404:bool)
                "Metronome Loop iteration" <- w392
              }
              n204 = call <vilib>:"Clear Errors.vi"("error in (no error)"=w42) -> ("error out"=w37:errorcluster)  [unwired: 5 in, 1 out]
              n205 = Merge Errors(w44, w46, w40, w38, w37) -> (w45:errorcluster)
            }
            frame Error {
              w413 = T18 1 items=["no dialog", "OK message", "continue or stop message", "OK message + warnings", "continue/stop + warnings"]  # Type of dialog
              # "Error during pre-loop initialisation. Exit VI."
              n206 = call <vilib>:"Simple Error Handler.vi"("type of dialog (OK msg:1)"=w413, "error in (no error)"=w415) -> ("error out"=w414:errorcluster)  [unwired: 3 in, 4 out]
            }
          }
        }
        frame Error {
          w418 = T18 1 items=["no dialog", "OK message", "continue or stop message", "OK message + warnings", "continue/stop + warnings"]  # Type of dialog
          n207 = call <vilib>:"Simple Error Handler.vi"("type of dialog (OK msg:1)"=w418, "error in (no error)"=w417) -> ("error out"=w416:errorcluster)  [unwired: 3 in, 4 out]
        }
      }
    }
    frame Error {
    }
  }
  "Error Out" <- w3
  n208 = disable-structure shown="Disabled" {
    frame Disabled {
      # "Commonly inspected VIs and typedefs"
    }
    frame Enabled {
    }
  }
